vi "svx_Colormap Get Edit-time Menu Label.vi"(11 "MenuRef":refnum<k9>) -> (1 "Disable item tags":string[](array[string])=["USER_SC_SCALE_LEGEND", "USER_SC_GRAPH_PALETTE", "USER_SC_CURSOR_LEGEND", "USER_SC_X_SCALE", "USER_SC_Y_SCALE", "USER_SC_Z_SCALE", "USER_SC_AUTOSCALE_X", "USER_SC_AUTOSCALE_Y", "USER_SC_AUTOSCALE_Z", "USER_SC_IGNORE_COLOR_ARRAY", "USER_SC_INTERPOLATE_COLOR", "USER_SC_SMOOTH_UPDATES", "USER_SC_LABEL", "USER_SC_CAPTION", "USER_SC_ORDER", "USER_SC_FREQ"], 2 "item tags":string[](array[string])=["USER_SC_SCALE_LEGEND", "USER_SC_GRAPH_PALETTE", "USER_SC_CURSOR_LEGEND", "USER_SC_X_SCALE", "USER_SC_Y_SCALE", "USER_SC_Z_SCALE", "USER_SC_AUTOSCALE_X", "USER_SC_AUTOSCALE_Y", "USER_SC_AUTOSCALE_Z", "USER_SC_IGNORE_COLOR_ARRAY", "USER_SC_INTERPOLATE_COLOR", "USER_SC_SMOOTH_UPDATES", "USER_SC_LABEL", "USER_SC_CAPTION", "USER_SC_ORDER", "USER_SC_FREQ"], 3 "menu reference out":refnum<k9>)   [LabVIEW 2017, in "SVX Colormap.xctl"]
uses:
  <vilib>/addons/_XControls/Colormap/SVX Colormap.xctl
panel:
  in  "menu items":T1(array[cluster])=[{"menu tag"="APP_SC_VISIBLE_ITEMS", "item names"="Label", "item tags"="USER_SC_LABEL", ""}, {"menu tag"="APP_SC_VISIBLE_ITEMS", "item names"="Caption", "item tags"="USER_SC_CAPTION", "USER_SC_LABEL"}, {"menu tag"="APP_SC_VISIBLE_ITEMS", "item names"="-", "item tags"="APP_SC_SEPERATOR", "USER_SC_CAPTION"}, {"menu tag"="APP_SC_VISIBLE_ITEMS", "item names"="Scale Legend", "item tags"="USER_SC_SCALE_LEGEND", "APP_SC_CAPTION"}, {"menu tag"="APP_SC_VISIBLE_ITEMS", "item names"="Graph Palette", "item tags"="USER_SC_GRAPH_PALETTE", "USER_SC_SCALE_LEGEND"}, {"menu tag"="APP_SC_VISIBLE_ITEMS", "item names"="Cursor Legend", "item tags"="USER_SC_CURSOR_LEGEND", "USER_SC_GRAPH_PALETTE"}, {"menu tag"="APP_SC_VISIBLE_ITEMS", "item names"="X Scale", "item tags"="USER_SC_X_SCALE", "USER_SC_CURSOR_LEGEND"}, {"menu tag"="APP_SC_VISIBLE_ITEMS", "item names"="Y Scale", "item tags"="USER_SC_Y_SCALE", "USER_SC_X_SCALE"}, {"menu tag"="APP_SC_VISIBLE_ITEMS", "item names"="Z Scale", "item tags"="USER_SC_Z_SCALE", "USER_SC_Y_SCALE"}, {"menu tag"="", "item names"="AutoScale X", "item tags"="USER_SC_AUTOSCALE_X", ""}, {"menu tag"="", "item names"="AutoScale Y", "item tags"="USER_SC_AUTOSCALE_Y", "USER_SC_AUTOSCALE_X"}, {"menu tag"="", "item names"="AutoScale Z", "item tags"="USER_SC_AUTOSCALE_Z", "USER_SC_AUTOSCALE_Y"}, {"menu tag"="", "item names"="Ignore Color Array", "item tags"="USER_SC_IGNORE_COLOR_ARRAY", "USER_SC_AUTOSCALE_Z"}, {"menu tag"="", "item names"="Interpolate Color", "item tags"="USER_SC_INTERPOLATE_COLOR", "USER_SC_IGNORE_COLOR_ARRAY"}, {"menu tag"="", "item names"="Smooth Updates", "item tags"="USER_SC_SMOOTH_UPDATES", "USER_SC_INTERPOLATE_COLOR"}, {"menu tag"="APP_SC_VISIBLE_ITEMS", "item names"="-", "item tags"="APP_SC_SEPARATOR", "APP_SC_CAPTION"}, {"menu tag"="APP_SC_VISIBLE_ITEMS", "item names"="-", "item tags"="APP_SC_SEPARATOR_2", "USER_SC_CURSOR_LEGEND"}, {"menu tag"="", "item names"="-", "item tags"="APP_SC_SEPARATOR_3", "USER_SC_SMOOTH_UPDATES"}, {"menu tag"="", "item names"="Cursor Lines", "item tags"="USER_SC_DISPLAY", "APP_SC_SEPARATOR_3"}, {"menu tag"="USER_SC_DISPLAY", "item names"="Show Current Order", "item tags"="USER_SC_ORDER", ""}, {"menu tag"="USER_SC_DISPLAY", "item names"="Show Current Frequency", "item tags"="USER_SC_FREQ", "USER_SC_ORDER"}, {"menu tag"="USER_SC_DISPLAY", "item names"="Anchor Current", "item tags"="USER_SC_ADD", ""}, {"menu tag"="USER_SC_DISPLAY", "item names"="-", "item tags"="APP_SC_SEPARATOR_4", "USER_SC_ADD"}, {"menu tag"="USER_SC_DISPLAY", "item names"="Customize...", "item tags"="USER_SC_CREATE_INDICATION_LINES", "APP_SC_SEPARATOR_4"}, {"menu tag"="", "item names"="-", "item tags"="APP_SC_SEPARATOR_5", "USER_SC_DISPLAY"}, {"menu tag"="", "item names"="Properties", "item tags"="USER_SC_PROPERTIES", "APP_SC_SEPARATOR_5"}]
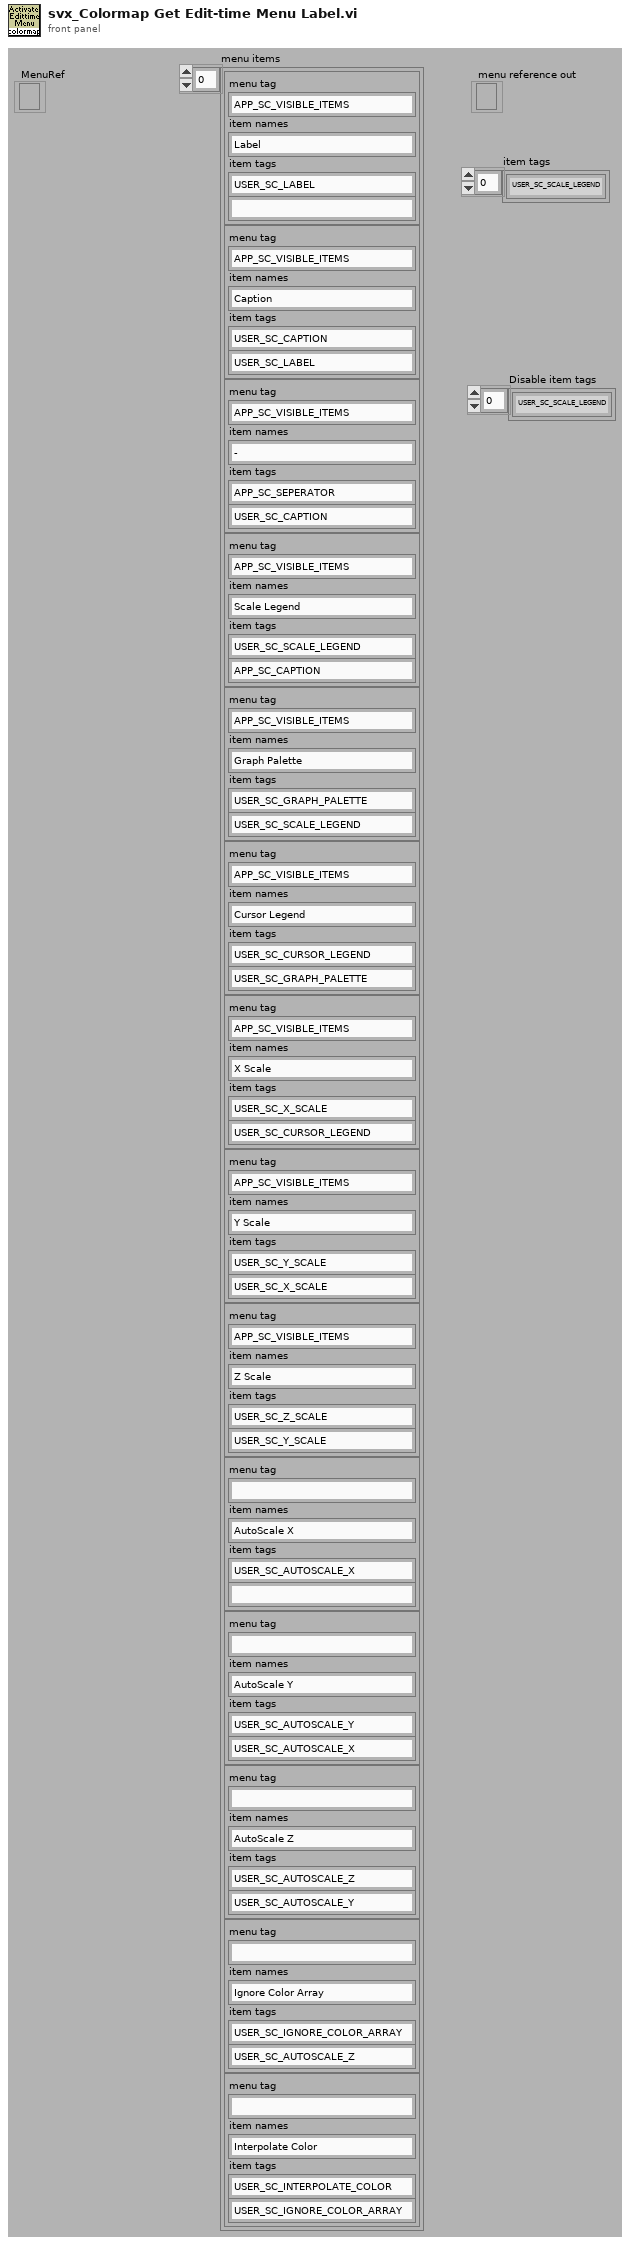
[diagram p1: front panel]
types:
  T1 = cluster{"menu tag":string, "item names":string, "item tags":string, string}[]
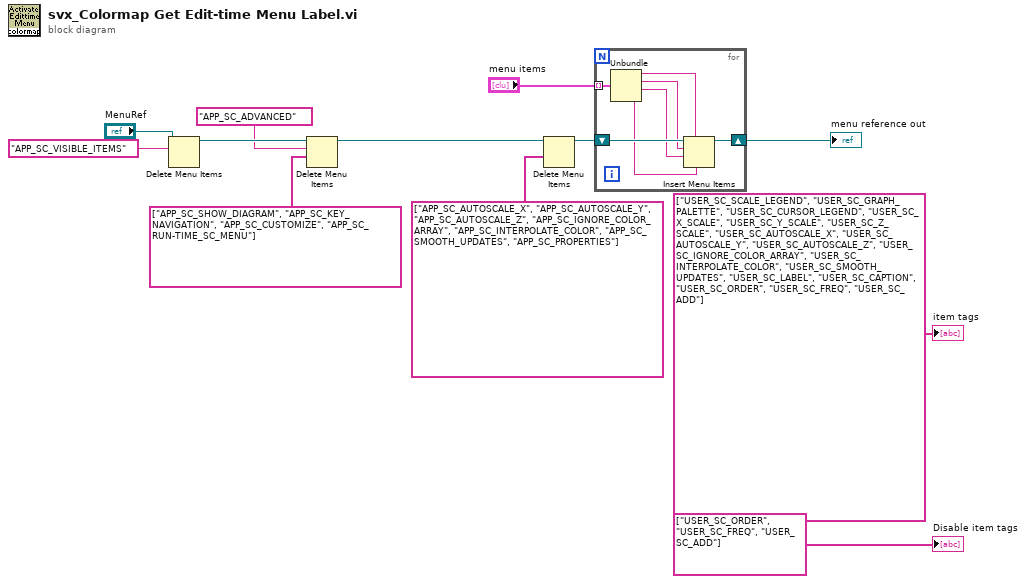
[diagram p0: block diagram]
diagram:
  n1 = Delete Menu Items(8:"APP_SC_VISIBLE_ITEMS", 9:"MenuRef") -> (3:w6:refnum<k9>)  [unwired: 2 in, 1 out]
  n2 = Delete Menu Items(7:string[] ["APP_SC_SHOW_DIAGRAM", "APP_SC_KEY_NAVIGATION", "APP_SC_CUSTOMIZE", "APP_SC_RUN-TIME_SC_MENU"] ("item tags"), 8:"APP_SC_ADVANCED", 9:w6) -> (3:w5:refnum<k9>)  [unwired: 1 in, 1 out]
  n3 = Delete Menu Items(7:string[] ["APP_SC_AUTOSCALE_X", "APP_SC_AUTOSCALE_Y", "APP_SC_AUTOSCALE_Z", "APP_SC_IGNORE_COLOR_ARRAY", "APP_SC_INTERPOLATE_COLOR", "APP_SC_SMOOTH_UPDATES", "APP_SC_PROPERTIES"] ("item tags"), 9:w5) -> (3:w9:refnum<k9>)  [unwired: 2 in, 1 out]
  n4 = for {
    shift-right: [w18] -> w2
    shift-left: w9 -> [w19]
    tunnel: "menu items" -> [w17] mode=indexing
    n5 = Unbundle(w17) -> ("menu tag"=w16:string, "item names"=w15:string, "item tags"=w14:string, w13:string)
    n6 = Insert Menu Items(4:w13, 5:w16, 7:w14, 8:w15, 9:w19) -> (3:w18:refnum<k9>)  [unwired: 1 in, 2 out]
  }
  "menu reference out" <- w2
  "item tags" <- string[] ["USER_SC_SCALE_LEGEND", "USER_SC_GRAPH_PALETTE", "USER_SC_CURSOR_LEGEND", "USER_SC_X_SCALE", "USER_SC_Y_SCALE", "USER_SC_Z_SCALE", "USER_SC_AUTOSCALE_X", "USER_SC_AUTOSCALE_Y", "USER_SC_AUTOSCALE_Z", "USER_SC_IGNORE_COLOR_ARRAY", "USER_SC_INTERPOLATE_COLOR", "USER_SC_SMOOTH_UPDATES", "USER_SC_LABEL", "USER_SC_CAPTION", "USER_SC_ORDER", "USER_SC_FREQ", "USER_SC_ADD"] ("item tags")
  "Disable item tags" <- string[] ["USER_SC_ORDER", "USER_SC_FREQ", "USER_SC_ADD"] ("Disable item tags")
